vi "DataPacker_Setup.vi"(5 "DataPacker Queue":refnum<queue>, 6 "Main VI Name":string, 8 "error in (no error)":errorcluster, 9 "Port To Log To":u16, 10 "Address to Log To":u32, 11 "DataPacker in":refnum<class "DataPacker.lvclass">) -> (0 "error out":errorcluster, 3 "DataPacker out":refnum<class "DataPacker.lvclass">)   [LabVIEW 2018, in "feGEM DataPacker.lvlib" / "DataPacker.lvclass"]
uses:
  DataPacker.lvclass
  DataStructures/GEM_BANK_CLUSTER_typedef.ctl
  DataStructures/GEM_DATA_cluster_typedef.ctl
  DataPacker.lvclass/DataPacker.ctl
  feGEM DataPacker.lvlib
  <vilib>/Utility/SystemLogging/NI_SystemLogging.lvlib
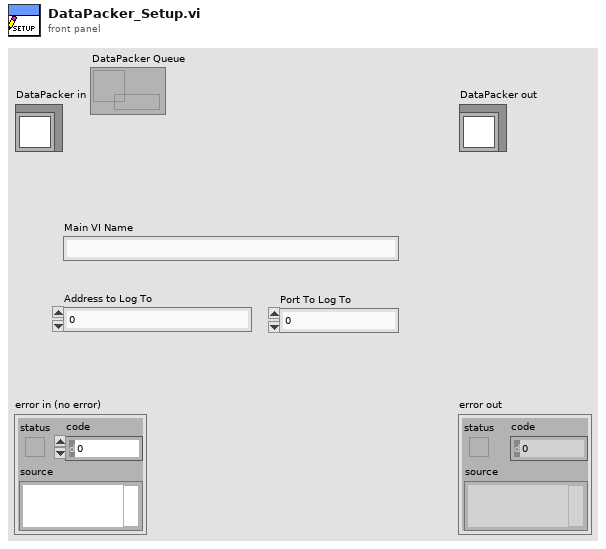
[diagram p1: front panel]
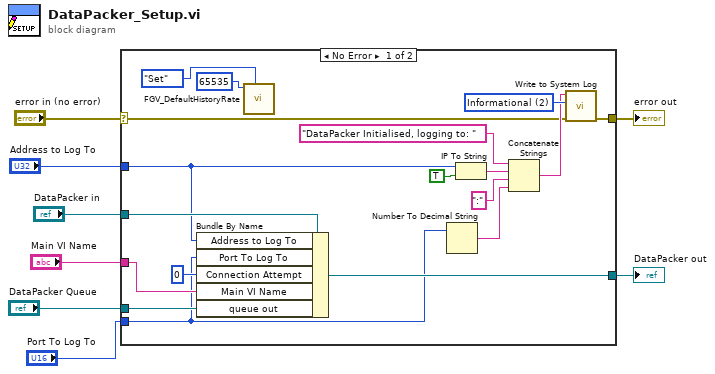
[diagram p0: block diagram]
diagram:
  n1 = case shown="No Error" "error in (no error)" {
    selector: "error in (no error)" -> [w10 w27]
    tunnel: [w9 w27] -> w7
    tunnel: [w26 w28] -> w5
    tunnel: "DataPacker in" -> [w21 w28]
    tunnel: "Port To Log To" -> [w13 _]
    tunnel: "Main VI Name" -> [w22 _]
    tunnel: "DataPacker Queue" -> [w20 _]
    tunnel: "Address to Log To" -> [w17 _]
    frame No Error {
      w19 = 2 items=["Error", "Warning", "Informational"] ("severity")
      n2 = Bundle By Name(cluster=w21, "Address to Log To"=w17, "Port To Log To"=w13, "Connection Attempt"=u32 0, "Main VI Name"=w22, "queue out"=w20) -> (w26:refnum<class "DataPacker.lvclass">)
      n3 = call "FGV_DefaultHistoryRate.vi"("Default History Rate"=65535, "Enum"=enum16{"Set", "Get"}."Set") -> ()  [unwired: 3 in, 1 out]
      n4 = Number To Decimal String(number=w13) -> (decimal integer string=w12:string)  [unwired: 1 in]
      n5 = IP To String(1:TRUE ("dot notation? (F)"), 2:w17) -> (0:w15:string)
      n6 = Concatenate Strings("DataPacker Initialised, logging to: " ("message"), w15, ":" ("string"), w12) -> (w11:string)
      n7 = call <vilib>:"Write to System Log.vi"("error in (no error)"=w10, "severity"=w19, "message"=w11) -> ("error out"=w9:errorcluster)  [unwired: 8 in]
    }
    frame Error {
    }
  }
  "error out" <- w7
  "DataPacker out" <- w5
